vi "V2FGV.vi"(8 "Error In":errorcluster, 10 "action(write)":enum16{"write", "read"}(ring), 11 "V2 in":dbl) -> (0 "Error Out":errorcluster, 3 "V2 out":dbl)   [LabVIEW 2020]
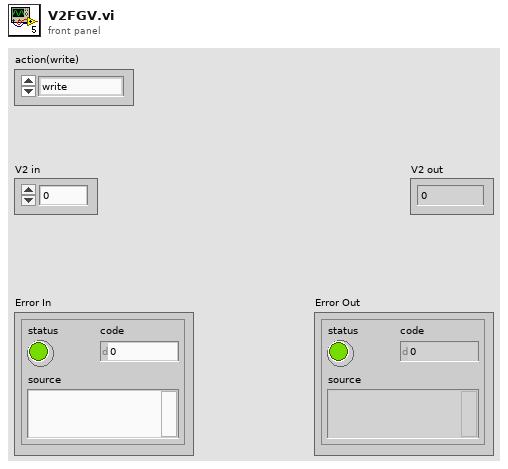
[diagram p1: front panel]
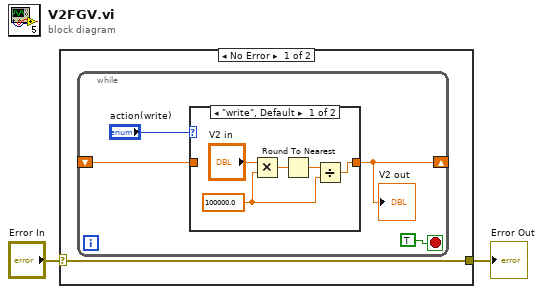
[diagram p0: block diagram]
diagram:
  n1 = case shown="No Error" "Error In" {
    selector: "Error In" -> [w3 w14]
    tunnel: [w3 w14] -> w1
    frame No Error {
      n2 = while {
        shift-right: [w6] -> _
        shift-left: _ -> [w4]
        stop <- TRUE stop-if-true
        n3 = case shown="\"write\", Default" "action(write)" {
          tunnel: [w8 w13] -> w6
          tunnel: w4 -> [_ w13]
          frame "write", Default {
            w9 = 100000.0 ("y")
            n4 = Multiply(x="V2 in", y=w9) -> (x*y=w11:dbl)
            n5 = Round To Nearest(number=w11) -> (nearest integer value=w10:dbl)
            n6 = Divide(x=w10, y=w9) -> (x/y=w8:dbl)
          }
          frame "read" {
          }
        }
        "V2 out" <- w6
      }
    }
    frame Error {
    }
  }
  "Error Out" <- w1
